vi "Power Supply Control Panel (No Objects).vi"(8 "error in (no error)":errorcluster) -> (0 "error out":errorcluster)   [LabVIEW 2009]
uses:
  Magnet status.ctl
  Oxford/PSSUBS.LLB/PSIO.ctl
  Oxford/BUSGEN.LLB/OxfordAddress.ctl
  Global/Relative Sound Files.vi
  Power Supply.lvclass
panel:
  out "*ips120 (No Ob)":T4={"Field"=0.0, "Rate"=0.0, "Status"={"Sweeping"=FALSE, "Clamped"=FALSE, "Hold"=FALSE, "At Rest"=FALSE, "Quench"=FALSE, "Persistent Mode"=FALSE, "Switch Heater"=FALSE}, "ILM Shut Down?"=FALSE, "IO Info"={"Address"={"Com Port"=1, "ISOBUS Address"=2, "GPIB Address"=24, "Communication"=enum."ISOBUS"}, "Version"=enum."IPS"}, "IO Info (Level Meter)"={"Address"={"Com Port"=1, "ISOBUS Address"=5, "GPIB Address"=24, "Communication"=enum."ISOBUS"}, "ILM Name"="", "Display Channel"=[]}, "Training?"=FALSE, "Training Field and Speed Cluster"={"Training Field"=[0.0, 4.108, 5.78, 8.001], "Training Speed"=[0.0057, 0.0022833333333333334, 0.0011333333333333334, 0.0011333333333333334]}}
  in  "Cluster In":T4={"Field"=0.0, "Rate"=0.0, "Status"={"Sweeping"=FALSE, "Clamped"=FALSE, "Hold"=FALSE, "At Rest"=FALSE, "Quench"=FALSE, "Persistent Mode"=FALSE, "Switch Heater"=FALSE}, "ILM Shut Down?"=FALSE, "IO Info"={"Address"={"Com Port"=1, "ISOBUS Address"=2, "GPIB Address"=24, "Communication"=enum."ISOBUS"}, "Version"=enum."IPS"}, "IO Info (Level Meter)"={"Address"={"Com Port"=1, "ISOBUS Address"=5, "GPIB Address"=24, "Communication"=enum."ISOBUS"}, "ILM Name"="", "Display Channel"=[]}, "Training?"=FALSE, "Training Field and Speed Cluster"={"Training Field"=[0.0, 4.108, 5.78, 8.001], "Training Speed"=[0.0057, 0.0022833333333333334, 0.0011333333333333334, 0.0011333333333333334]}}
  out "Was at persistent?":bool
  in  "Return to persistent?":bool
  out "log counter":dbl
  out "Going to Field?":bool
  out "Current Field":dbl[unit]
  out "Update UI":bool
  out "Status":T1
  in  "Abort Field Sweep":bool
  out "done?":bool
  out "ILM Shut Down?":bool
  out "SH On":bool caption="Switch Heater"
  out "Persistent Mode":bool
  in  "SHcontrol":bool caption="Switch Heater"
  in  "gotopersistent":bool
  out "active":bool
  in  "Train\nMagnet":bool
  out "Busy":bool
  out "ready?":bool
  in  "rate":dbl[unit]=0.016666666666666666 caption="Rate" min=0.0 max=0.25
  in  "Goto":dbl[unit]
  in  "Clamp":bool
  in  "Check for Magnet":bool
  in  "Hold":bool
  in  "Goto Zero":bool
  in  "Goto Field":bool
  in  "endprgm":bool
  # "Magnet Control Panel"
  # "(at current field)"
  # "Off"
  # "On"
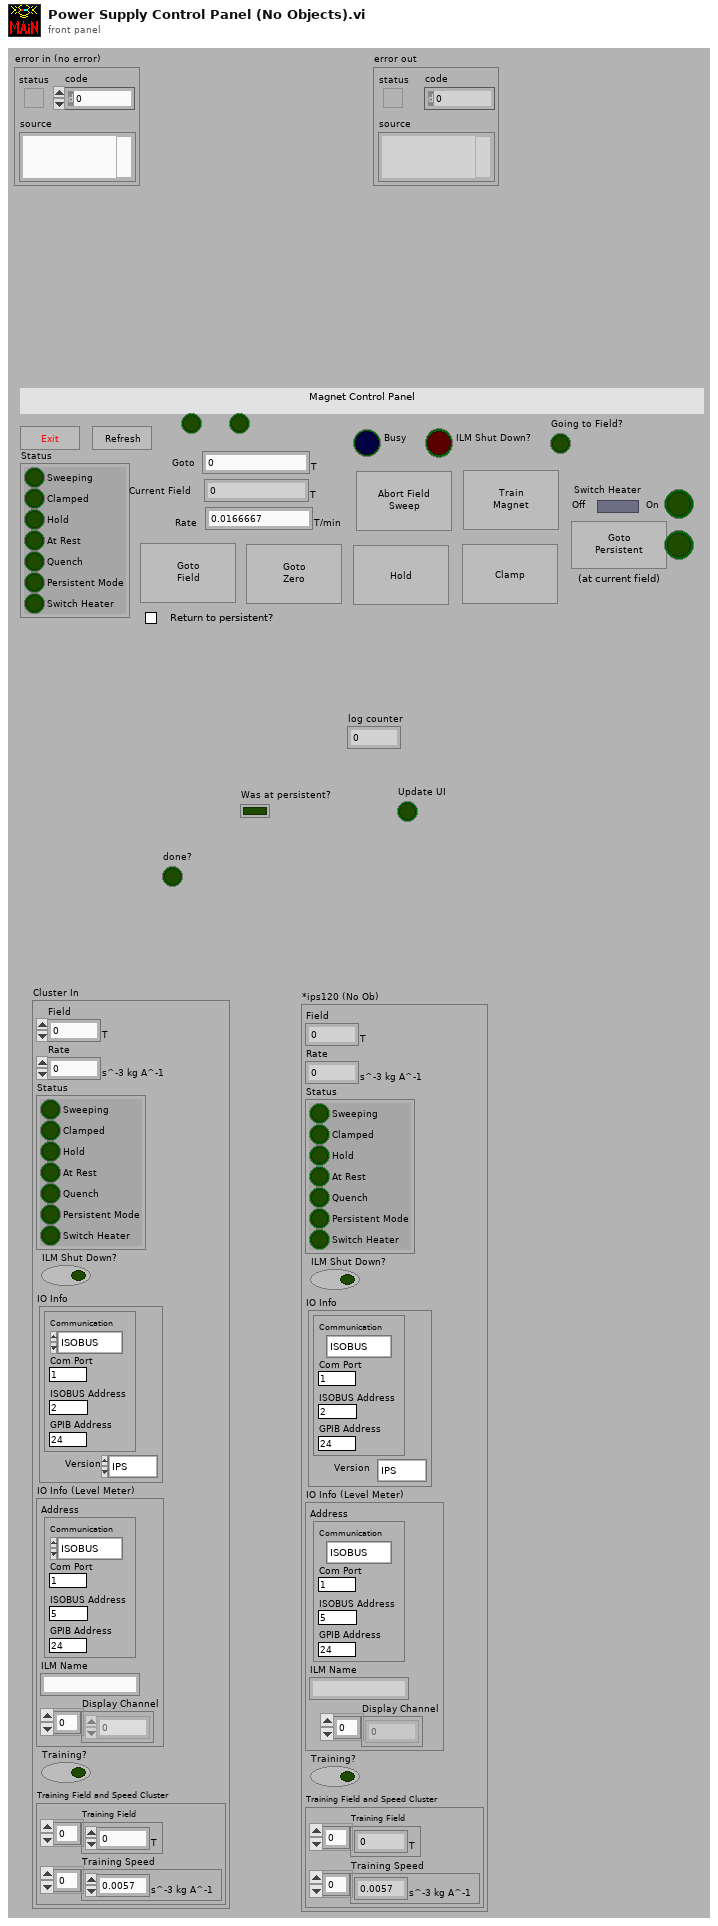
[diagram p1: front panel]
types:
  T1 = typedef "Power Supply.lvclass/Magnet status.ctl" = cluster{"Sweeping":bool, "Clamped":bool, "Hold":bool, "At Rest":bool, "Quench":bool, "Persistent Mode":bool, "Switch Heater":bool}
  T2 = typedef "PSIO.ctl" = cluster{"Address":T3, "Version":enum16{"PS", "IPS"}}
  T3 = typedef "OxfordAddress.ctl" = cluster{"Com Port":i32, "ISOBUS Address":i32, "GPIB Address":i16, "Communication":enum16{"RS232", "ISOBUS", "GPIB", "Gateway"}}
  T4 = cluster{"Field":dbl[unit], "Rate":dbl[unit], "Status":T1, "ILM Shut Down?":bool, "IO Info":T2, "IO Info (Level Meter)":cluster{"Address":T3, "ILM Name":string, "Display Channel":i32[]}, "Training?":bool, "Training Field and Speed Cluster":cluster{"Training Field":dbl[unit][], "Training Speed":dbl[unit][]}}
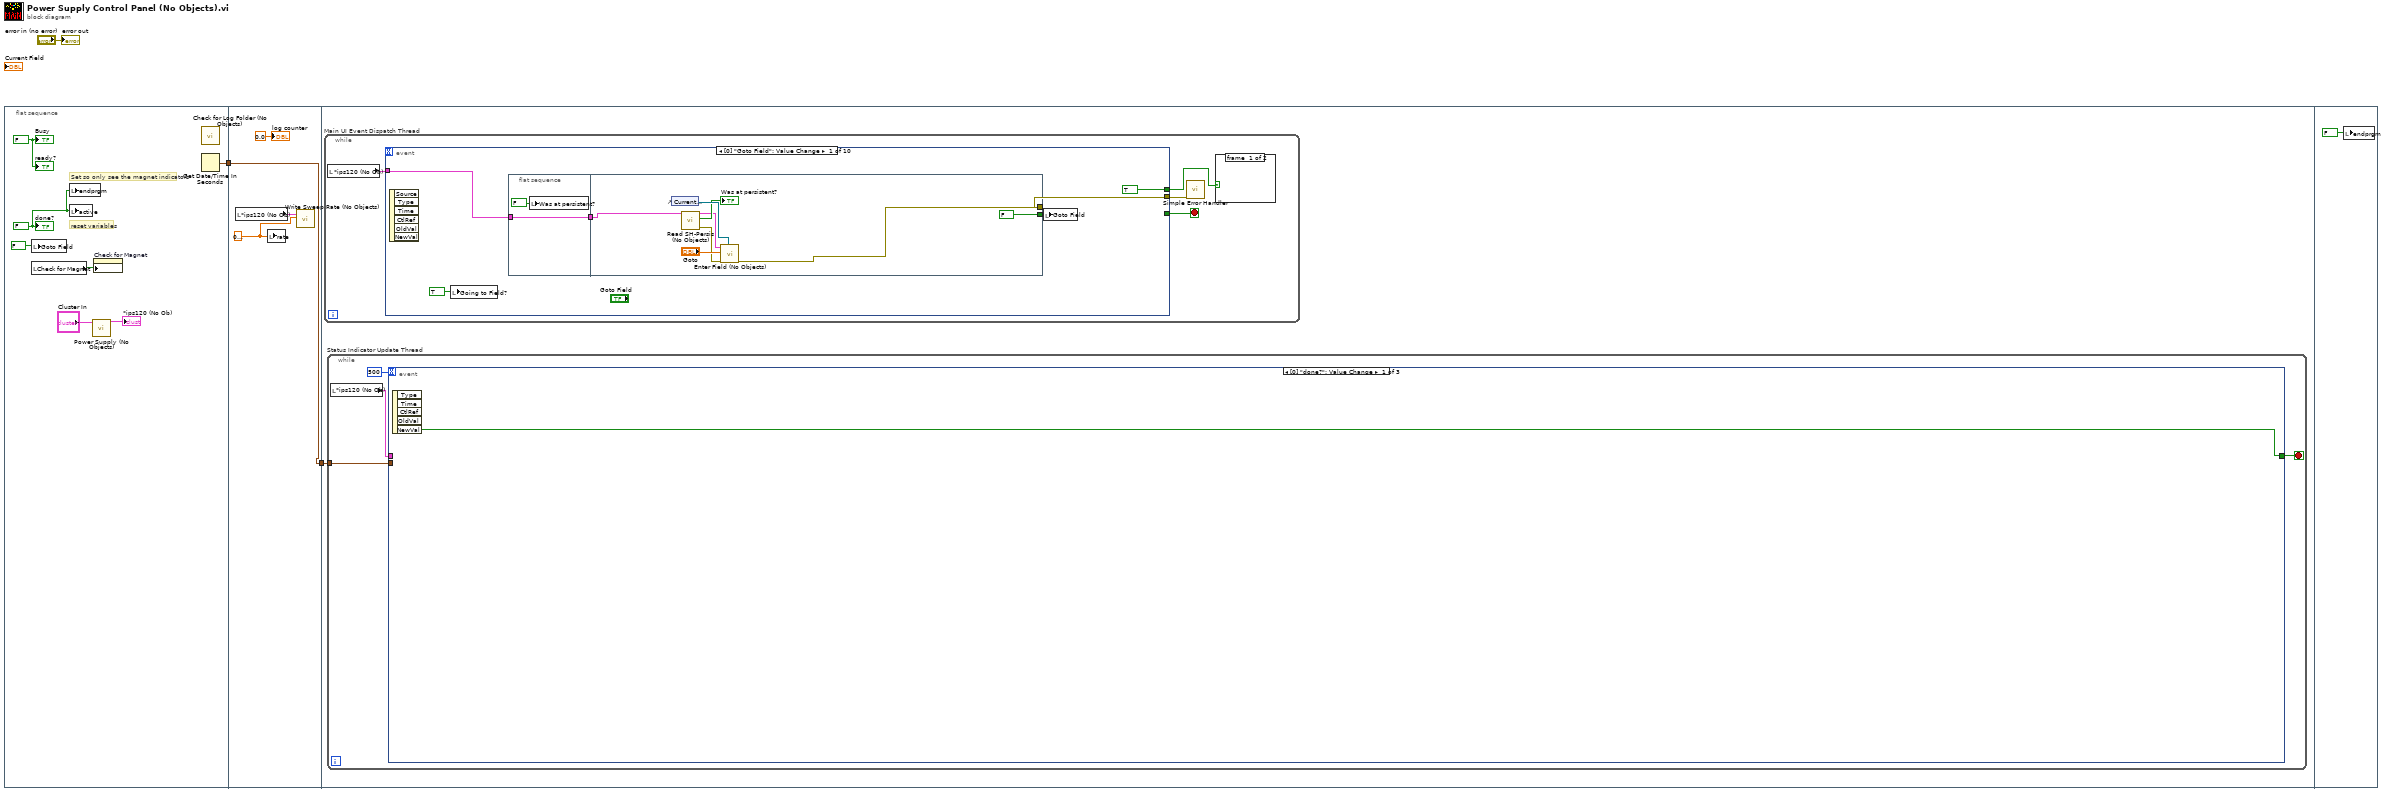
[diagram p0: block diagram]
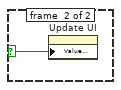
[diagram p2: hidden frame]
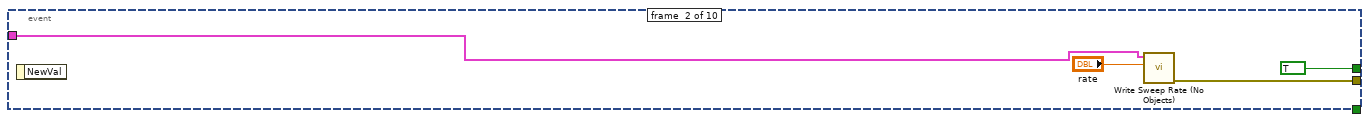
[diagram p3: hidden frame]
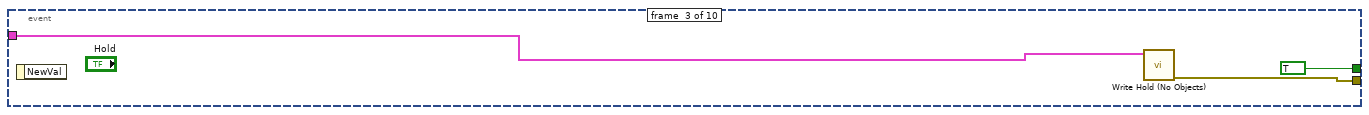
[diagram p4: hidden frame]
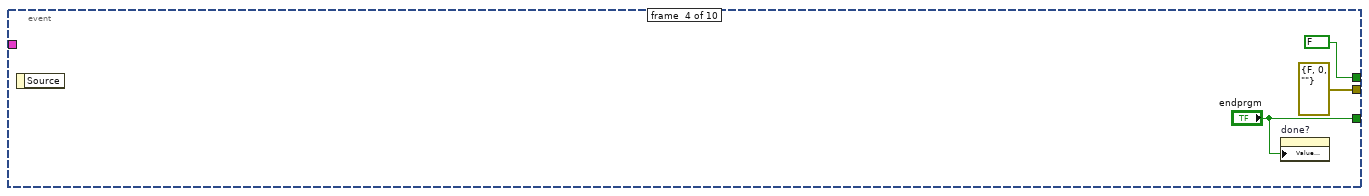
[diagram p5: hidden frame]
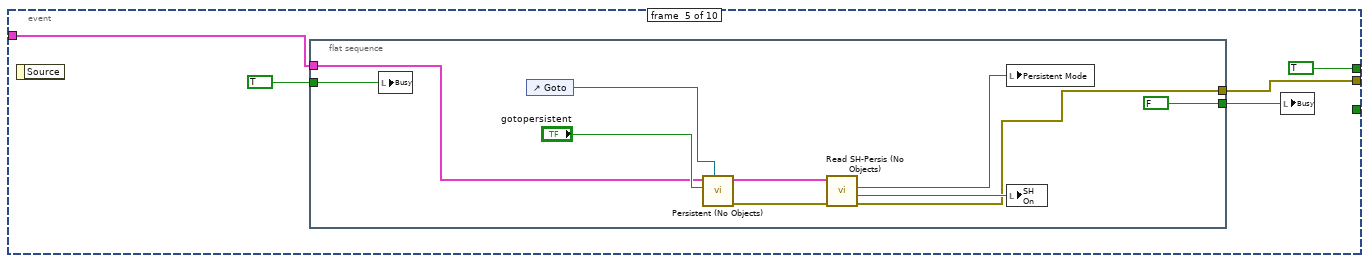
[diagram p6: hidden frame]
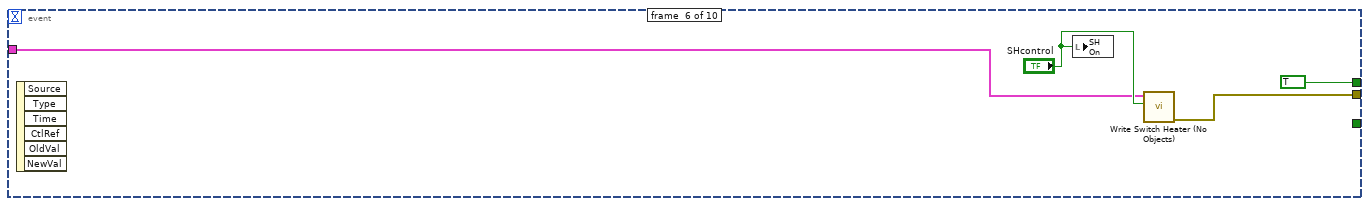
[diagram p7: hidden frame]
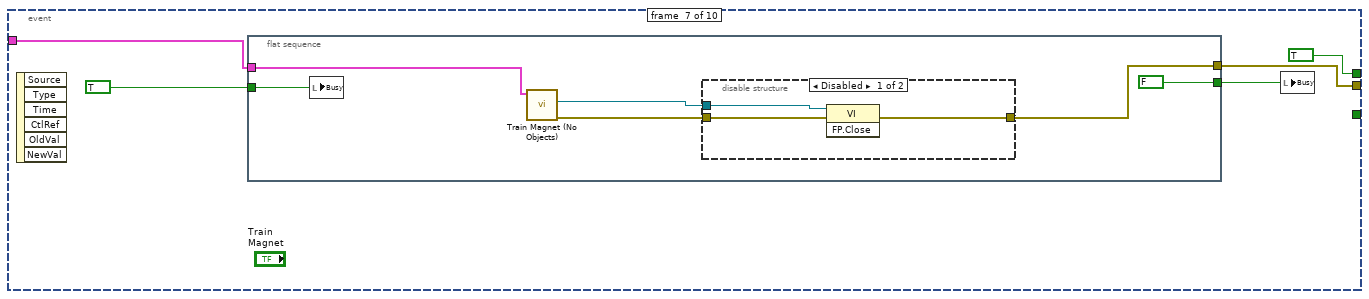
[diagram p8: hidden frame]
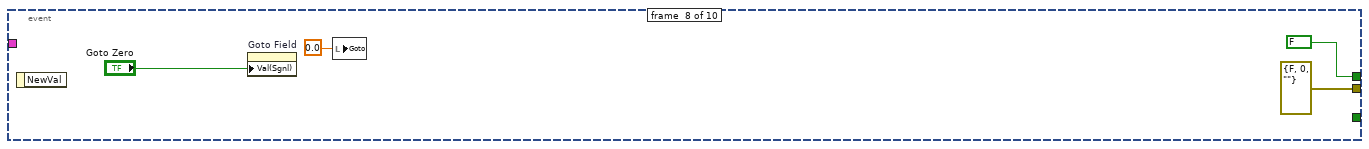
[diagram p10: hidden frame]
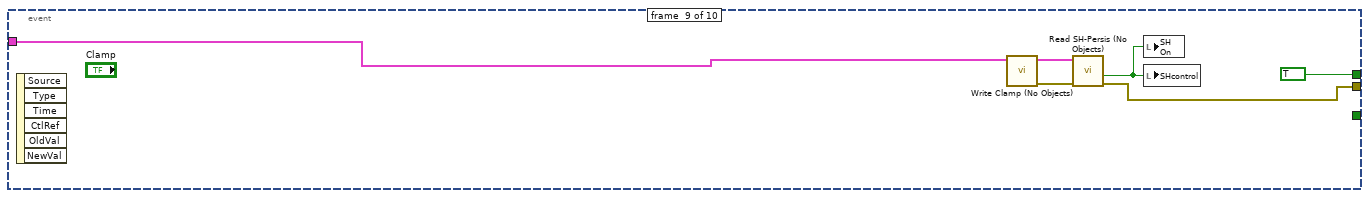
[diagram p11: hidden frame]
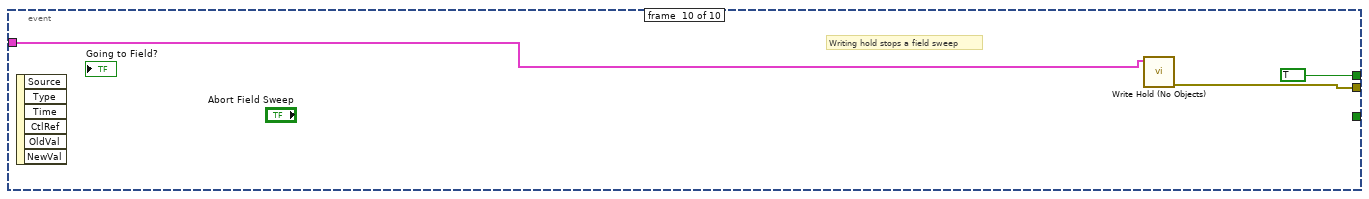
[diagram p12: hidden frame]
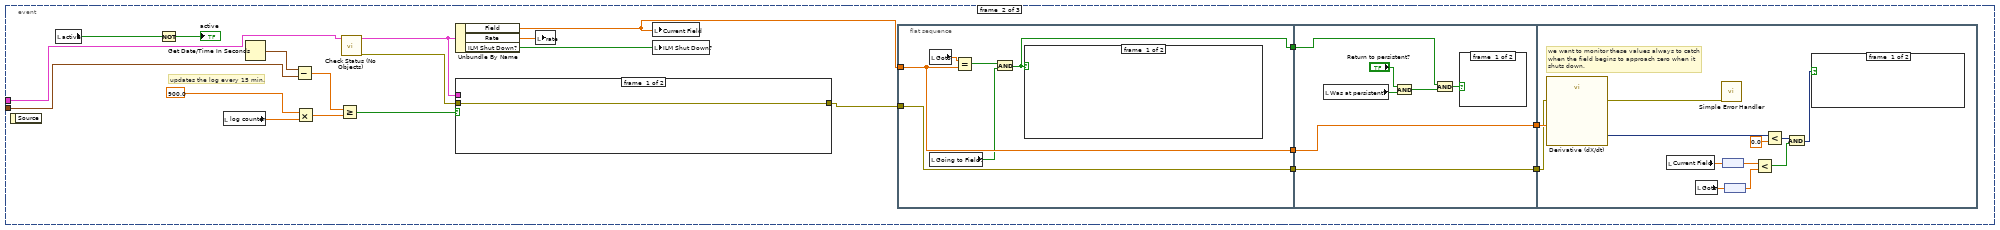
[diagram p13: hidden frame]
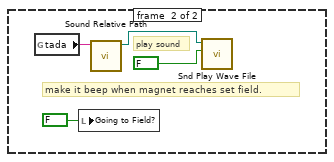
[diagram p14: hidden frame]
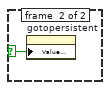
[diagram p15: hidden frame]
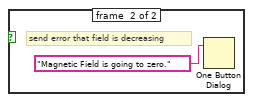
[diagram p16: hidden frame]
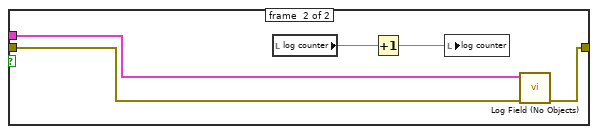
[diagram p17: hidden frame]
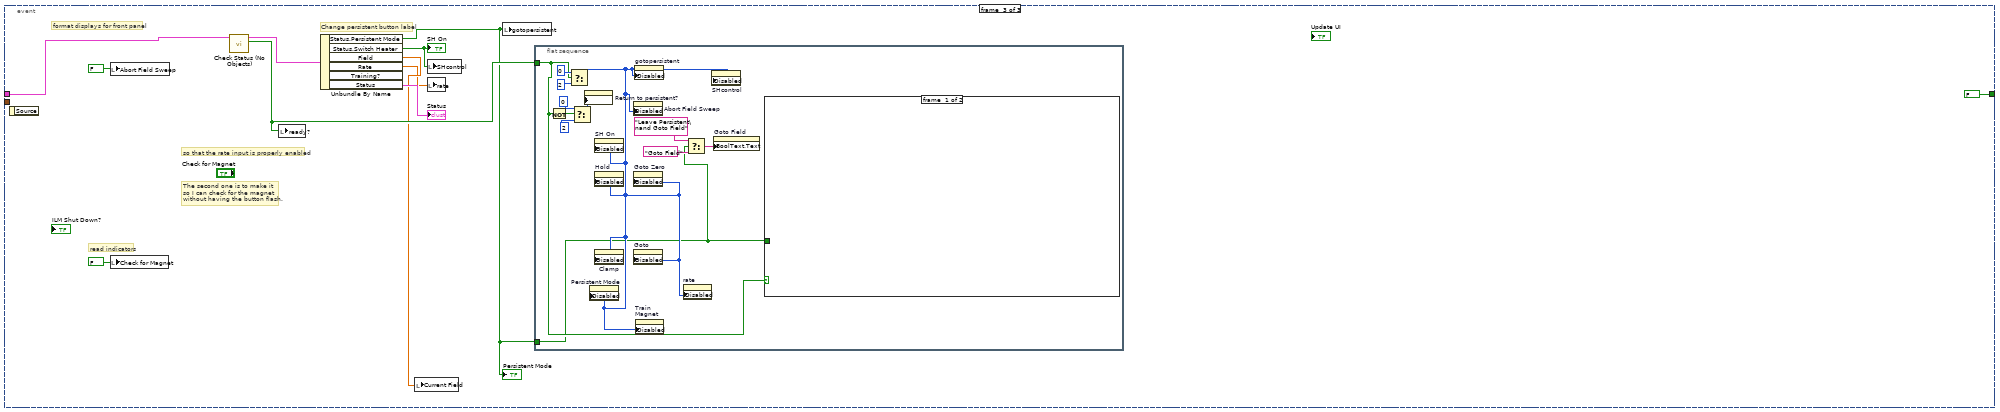
[diagram p18: hidden frame]
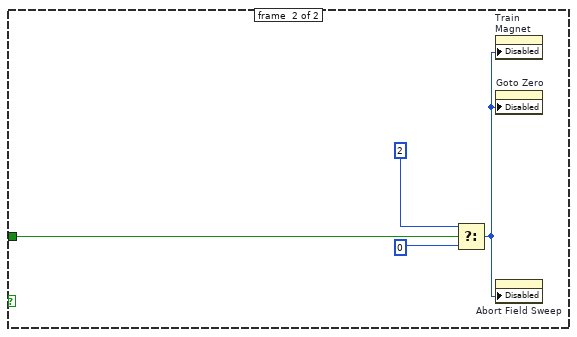
[diagram p19: hidden frame]
diagram:
  n1 = flat-sequence {
    tunnel: [w6] -> w2
    tunnel: w2 -> [w11]
    tunnel: [w11] -> w1
    tunnel: w1 -> [w15]
    frame #0 {
      w10 = FALSE
      w8 = FALSE
      # "Set so only see the magnet indicators"
      # "reset variables"
      n2 = local read "Check for Magnet"() -> (w9:bool)
      n3 = local write "Goto Field"(FALSE ("active")) -> ()
      n4 = local write "endprgm"(w8) -> ()
      n5 = local write "active"(w8) -> ()
      n6 = call "Power Supply (No Objects).vi"("Cluster In"="Cluster In") -> ("Cluster Out"=→"*ips120 (No Ob)":T4)  [unwired: 9 in, 1 out]
      n7 = property on="Check for Magnet" class="Bool (strict)"("Value (Signaling)"=w9) -> ()  [unwired: 2 in, 2 out]
      n8 = call "Check for Log Folder (No Objects).vi"() -> ()  [unwired: 1 in]
      n9 = Get Date/Time In Seconds() -> (seconds since 1Jan1904=w6:timestamp)
      "ready?" <- w10
      "Busy" <- w10
      "done?" <- w8
    }
    frame #1 {
      w12 = dbl[unit] 0.016666666666666666 ("rate")
      n10 = local read "*ips120 (No Ob)"() -> (w13:T4)
      n11 = local write "rate"(w12) -> ()
      n12 = call "Write Sweep Rate (No Objects).vi"("rate"=w12, "Cluster In"=w13) -> ()  [unwired: 8 in, 2 out]
      "log counter" <- 0.0 ("log counter")
    }
    frame #2 {
      n13 = while "Main UI Event Dispatch Thread" {
        stop <- w18 stop-if-true
        n14 = local read "*ips120 (No Ob)"() -> (w16:T4)
        n15 = event shown="[0] \"Goto Field\": Value Change" {
          selector: _ -> [_ _ _ _ _ _ _ _ _ _]
          dyn-events: _ -> [_ _ _ _ _ _ _ _ _ _]
          timeout: _ -> [_ _ _ _ _ _ _ _ _ _]
          tunnel: [_ _ _ "endprgm" _ _ _ _ _ _] -> w18
          tunnel: w16 -> [w26 w38 w41 _ w51 w62 w70 _ w86 w91]
          tunnel: [w24 w37 w42 errorcluster {"status"=FALSE, "code"=0, "source"=""} ("error out") w50 w63 w69 errorcluster {"status"=FALSE, "code"=0, "source"=""} ("error out") w87 w92] -> w19
          tunnel: [TRUE TRUE TRUE FALSE TRUE TRUE TRUE FALSE TRUE TRUE] -> w17
          event #0 {
            n16 = event-data() -> ()  [unwired: 7 out]
            n17 = local write "Going to Field?"(TRUE ("Going to Field?")) -> ()
            n18 = flat-sequence {
              tunnel: w26 -> [w28]
              tunnel: [w28] -> w21
              tunnel: [FALSE ("Goto Field")] -> w25
              tunnel: [w31] -> w24
              tunnel: w21 -> [w30]
              frame #0 {
                n19 = local write "Was at persistent?"(FALSE ("Was at persistent?")) -> ()
              }
              frame #1 {
                n20 = control-ref of="Current Field"() -> (w35:refnum<vi>)
                n21 = call "Read SH-Persis (No Objects).vi"("Cluster In"=w30) -> ("error out"=w33:errorcluster, "pers?"=→"Was at persistent?":bool, "Cluster Out"=w29:T4)  [unwired: 5 in, 3 out]
                n22 = call "Enter Field (No Objects).vi"("Field monitor"=w35, "error in (no error)"=w33, "Target field"="Goto", "Cluster In"=w29) -> ("error out"=w31:errorcluster)  [unwired: 6 in, 1 out]
              }
            }
            n23 = local write "Goto Field"(w25) -> ()
          }
          event #1 {
            n24 = event-data() -> ()  [unwired: 2 out]
            n25 = call "Write Sweep Rate (No Objects).vi"("rate"="rate", "Cluster In"=w38) -> ("error out"=w37:errorcluster)  [unwired: 8 in, 1 out]
          }
          event #2 {
            n26 = event-data() -> ()  [unwired: 2 out]
            n27 = call "Write Hold (No Objects).vi"("Cluster In"=w41) -> ("error out"=w42:errorcluster)  [unwired: 9 in, 1 out]
          }
          event #3 {
            n28 = event-data() -> ()  [unwired: 2 out]
            n29 = property on="done?" class="Boolean (strict)"("Value (Signaling)"="endprgm") -> ()  [unwired: 2 in, 2 out]
          }
          event #4 {
            n30 = event-data() -> ()  [unwired: 2 out]
            n31 = flat-sequence {
              tunnel: w51 -> [w53]
              tunnel: [w54] -> w50
              tunnel: TRUE -> [w56]
              tunnel: [FALSE] -> w47
              frame #0 {
                n32 = local write "Busy"(w56) -> ()
                n33 = control-ref of="Goto"() -> (w60:refnum<vi>)
                n34 = call "Persistent (No Objects).vi"("Field monitor ref"=w60, "Go to persistent mode?"="gotopersistent", "Cluster In"=w53) -> ("error out"=w61:errorcluster, "Cluster Out"=w52:T4)  [unwired: 7 in]
                n35 = call "Read SH-Persis (No Objects).vi"("error in (no error)"=w61, "Cluster In"=w52) -> ("error out"=w54:errorcluster, "SHon?"=w57:bool, "pers?"=w58:bool)  [unwired: 4 in, 3 out]
                n36 = local write "Persistent Mode"(w58) -> ()
                n37 = local write "SH On"(w57) -> ()
              }
            }
            n38 = local write "Busy"(w47) -> ()
          }
          event #5 {
            n39 = event-data() -> ()  [unwired: 7 out]
            n40 = local write "SH On"("SHcontrol") -> ()
            n41 = call "Write Switch Heater (No Objects).vi"("Turn SH On?"="SHcontrol", "Cluster In"=w62) -> ("error out"=w63:errorcluster)  [unwired: 8 in, 1 out]
          }
          event #6 {
            n42 = event-data() -> ()  [unwired: 7 out]
            n43 = flat-sequence {
              tunnel: w70 -> [w71]
              tunnel: [w72] -> w69
              tunnel: [FALSE] -> w67
              tunnel: TRUE -> [w75]
              frame #0 {
                n44 = local write "Busy"(w75) -> ()
                n45 = call "Train Magnet (No Objects).vi"("Cluster In"=w71) -> ("error out"=w73:errorcluster, "This VI"=w74:refnum<vi>)  [unwired: 8 in, 1 out]
                n46 = disable-structure shown="Disabled" {
                  disable-tunnel: w74 -> [w79 _]
                  disable-tunnel: w73 -> [w78 w80]
                  disable-tunnel: [w77 w80] -> w72
                  frame #0 {
                    n47 = invoke class="VI" method="FP.Close"(reference=w79, error in=w78) -> (error out=w77:errorcluster)  [unwired: 1 in, 2 out]
                  }
                  frame #1 {
                  }
                }
              }
            }
            n48 = local write "Busy"(w67) -> ()
          }
          event #7 {
            n49 = event-data() -> ()  [unwired: 2 out]
            n50 = property on="Goto Field" class="Bool (strict)"("Val(Sgnl)"="Goto Zero") -> ()  [unwired: 2 in, 2 out]
            n51 = local write "Goto"(dbl[unit] 0.0 ("Goto")) -> ()
          }
          event #8 {
            n52 = event-data() -> ()  [unwired: 7 out]
            n53 = call "Write Clamp (No Objects).vi"("Cluster In"=w86) -> ("error out"=w90:errorcluster, "Cluster Out"=w85:T4)  [unwired: 9 in]
            n54 = call "Read SH-Persis (No Objects).vi"("error in (no error)"=w90, "Cluster In"=w85) -> ("error out"=w87:errorcluster, "SHon?"=w89:bool)  [unwired: 4 in, 4 out]
            n55 = local write "SH On"(w89) -> ()
            n56 = local write "SHcontrol"(w89) -> ()
          }
          event #9 {
            # "Writing hold stops a field sweep"
            n57 = event-data() -> ()  [unwired: 7 out]
            n58 = call "Write Hold (No Objects).vi"("Cluster In"=w91) -> ("error out"=w92:errorcluster)  [unwired: 9 in, 1 out]
          }
        }
        n59 = call <vilib>:"Simple Error Handler.vi"("error in (no error)"=w19) -> ()  [unwired: 4 in, 5 out]
        n60 = case shown="True" w17 {
          selector: w17 -> [_ w20]
          frame #0 {
          }
          frame #1 {
            n61 = property on="Update UI" class="Bool (strict)"("Value (Signaling)"=w20) -> ()  [unwired: 2 in, 2 out]
          }
        }
      }
      n62 = while "Status Indicator Update Thread" {
        tunnel: w15 -> [w95]
        stop <- w96 stop-if-true
        n63 = local read "*ips120 (No Ob)"() -> (w94:T4)
        n64 = event shown="[0] \"done?\": Value Change" {
          selector: _ -> [_ _ _]
          dyn-events: _ -> [_ _ _]
          timeout: 500 -> [_ _ _]
          tunnel: [w98 _ FALSE] -> w96
          tunnel: w94 -> [_ w100 w157]
          tunnel: w95 -> [_ w117 _]
          event #0 {
            n65 = event-data() -> ("NewVal"=w98:bool)  [unwired: 5 out]
          }
          event #1 {
            # "updates the log every 15 min."
            n66 = event-data() -> ()  [unwired: 2 out]
            n67 = local read "active"() -> (w119:bool)
            n68 = Not(x=w119) -> (.not. x?=→"active":bool)
            n69 = local read "log counter"() -> (w108:dbl)
            n70 = Get Date/Time In Seconds() -> (seconds since 1Jan1904=w111:timestamp)
            n71 = Subtract(x=w111, y=w117) -> (x-y=w106:dbl)
            n72 = Multiply(x=900.0 ("millisecond multiple"), y=w108) -> (x*y=w107:dbl)
            n73 = Greater Or Equal?(x=w106, y=w107) -> (x >= y?=w112:bool)
            n74 = call "Check Status (No Objects).vi"("Cluster In"=w100) -> ("error out"=w113:errorcluster, "Cluster Out"=w114:T4)  [unwired: 7 in, 2 out]
            n75 = Unbundle By Name(w114) -> ("Field"=w115:dbl[unit], "Rate"=w110:dbl[unit], "ILM Shut Down?"=w116:bool)
            n76 = case shown="True" w112 {
              tunnel: [w151 w156] -> w99
              tunnel: w114 -> [_ w152]
              tunnel: w113 -> [w151 w155]
              frame #0 {
              }
              frame #1 {
                n77 = local read "log counter"() -> (w154:dbl)
                n78 = Increment(x=w154) -> (x+1=w153:dbl)
                n79 = local write "log counter"(w153) -> ()
                n80 = call "Log Field (No Objects).vi"("error in (no error)"=w155, "Cluster In"=w152) -> ("error out"=w156:errorcluster)  [unwired: 8 in, 1 out]
              }
            }
            n81 = local write "rate"(w110) -> ()
            n82 = local write "Current Field"(w115) -> ()
            n83 = local write "ILM Shut Down?"(w116) -> ()
            n84 = flat-sequence {
              tunnel: w99 -> [w125]
              tunnel: w115 -> [w123]
              tunnel: [w123] -> w105
              tunnel: [w125] -> w104
              tunnel: [w120] -> w103
              tunnel: w105 -> [w136]
              tunnel: [w136] -> w102
              tunnel: w104 -> [w135]
              tunnel: [w135] -> w101
              tunnel: w103 -> [w133]
              tunnel: w102 -> [w149]
              tunnel: w101 -> [w148]
              frame #0 {
                n85 = local read "Goto"() -> (w124:dbl[unit])
                n86 = local read "Going to Field?"() -> (w121:bool)
                n87 = Equal?(x=w124, y=w123) -> (x = y?=w122:bool)
                n88 = And(x=w122, y=w121) -> (x .and. y?=w120:bool)
                n89 = case shown="True" w120 {
                  frame #0 {
                  }
                  frame #1 {
                    # "make it beep when magnet reaches set field."
                    # "play sound"
                    n90 = global read "Relative Sound Files.vi" "tada"() -> (w127:string)
                    n91 = local write "Going to Field?"(FALSE ("Going to Field?")) -> ()
                    n92 = call "Sound Relative Path.vi"("Sound"=w127) -> ("Relative Path"=w128:path)  [unwired: 10 in]
                    n93 = call <vilib>:"Snd Play Wave File.vi"("wait until finish (T)"=FALSE, "wave file path"=w128) -> ()  [unwired: 1 in, 9 out]
                  }
                }
              }
              frame #1 {
                n94 = local read "Was at persistent?"() -> (w132:bool)
                n95 = And(x="Return to persistent?", y=w132) -> (x .and. y?=w130:bool)
                n96 = And(x=w133, y=w130) -> (x .and. y?=w134:bool)
                n97 = case shown="True" w134 {
                  selector: w134 -> [_ w137]
                  frame #0 {
                  }
                  frame #1 {
                    n98 = property on="gotopersistent" class="Bool (strict)"("Value (Signaling)"=w137) -> ()  [unwired: 2 in, 2 out]
                  }
                }
              }
              frame #2 {
                # "we want to monitor these values always to catch\nwhen the field begins to approach zero when it\nshuts down."
                n99 = call "Derivative (dX/dt)"("error in (no error)"=w148, "Signals"=w149) -> ("error out"=w143:errorcluster, "Result"=w147:dynamicdata)  [unwired: 4 out]
                n100 = local read "Current Field"() -> (w139:dbl[unit])
                n101 = local read "Goto"() -> (w141:dbl[unit])
                n102 = call <vilib>:"Simple Error Handler.vi"("error in (no error)"=w143) -> ()  [unwired: 4 in, 5 out]
                n103 = node(w139) -> (w138:dbl)
                n104 = node(w141) -> (w140:dbl)
                n105 = Less?(x=w138, y=w140) -> (x < y?=w142:bool)
                n106 = Less?(x=w147, y=0.0) -> (x < y?=w145:dynamicdata)
                n107 = And(x=w145, y=w142) -> (x .and. y?=w144:dynamicdata)
                n108 = case shown="True" w144 {
                  frame #0 {
                  }
                  frame #1 {
                    # "send error that field is decreasing"
                    n109 = One Button Dialog(message="Magnetic Field is going to zero.") -> ()  [unwired: 1 in, 1 out]
                  }
                }
              }
            }
          }
          event #2 {
            # "format displays for front panel"
            # "read indicators"
            # "so that the rate input is properly enabled"
            # "Change persistent button label"
            # "The second one is to make it\nso I can check for the magnet\nwithout having the button flash."
            n110 = event-data() -> ()  [unwired: 2 out]
            n111 = local write "Abort Field Sweep"(FALSE ("Abort Field Sweep")) -> ()
            n112 = local write "Check for Magnet"(FALSE) -> ()
            n113 = call "Check Status (No Objects).vi"("Cluster In"=w157) -> ("Ready?"=w165:bool, "Cluster Out"=w163:T4)  [unwired: 7 in, 2 out]
            n114 = local write "ready?"(w165) -> ()
            n115 = Unbundle By Name(w163) -> ("Status.Persistent Mode"=w160:bool, "Status.Switch Heater"=w164:bool, "Field"=w161:dbl[unit], "Rate"=w158:dbl[unit], "Status"=→"Status":T1)  [unwired: 1 out]
            "Persistent Mode" <- w160
            "SH On" <- w164
            n116 = local write "Current Field"(w161) -> ()
            n117 = local write "SHcontrol"(w164) -> ()
            n118 = local write "rate"(w158) -> ()
            n119 = local write "gotopersistent"(w160) -> ()
            n120 = flat-sequence {
              tunnel: w160 -> [w168]
              tunnel: w165 -> [w174]
              frame #0 {
                n121 = Not(x=w174) -> (.not. x?=w173:bool)
                n122 = Select(t=0, s=w174, f=2) -> (s? t:f=w177:i32)
                n123 = Select(t=0, s=w173, f=2) -> (s? t:f=w172:i32)
                n124 = property on="Return to persistent?" class="Bool (strict)"("DisabledEnum"=w172) -> ()  [unwired: 2 in, 2 out]
                n125 = property on="Persistent Mode" class="Boolean (strict)"("Disabled"=w177) -> ()  [unwired: 2 in, 2 out]
                n126 = property on="SH On" class="Boolean (strict)"("Disabled"=w177) -> ()  [unwired: 2 in, 2 out]
                n127 = property on="Hold" class="Boolean"("Disabled"=w177) -> ()  [unwired: 2 in, 2 out]
                n128 = property on="Clamp" class="Boolean"("Disabled"=w177) -> ()  [unwired: 2 in, 2 out]
                n129 = property on="Abort Field Sweep" class="Bool (strict)"("Disabled"=w177) -> ()  [unwired: 2 in, 2 out]
                n130 = property on="Goto Zero" class="Bool"("Disabled"=w177) -> ()  [unwired: 2 in, 2 out]
                n131 = property on="Goto" class="DigNum (strict)"("Disabled"=w177) -> ()  [unwired: 2 in, 2 out]
                n132 = property on="gotopersistent" class="Bool (strict)"("Disabled"=w177) -> ()  [unwired: 2 in, 2 out]
                n133 = property on="Train\nMagnet" class="Boolean"("Disabled"=w177) -> ()  [unwired: 2 in, 2 out]
                n134 = property on="rate" class="DigNum (strict)"("Disabled"=w177) -> ()  [unwired: 2 in, 2 out]
                n135 = Select(t="Leave Persistent\nand Goto Field", s=w168, f="Goto Field") -> (s? t:f=w170:string)
                n136 = property on="SHcontrol" class="Boolean (strict)"("Disabled"=w177) -> ()  [unwired: 2 in, 2 out]
                n137 = property on="Goto Field" class="Bool (strict)"("BoolText.Text"=w170) -> ()  [unwired: 2 in, 2 out]
                n138 = case shown="True" w174 {
                  tunnel: w168 -> [_ w181]
                  frame #0 {
                  }
                  frame #1 {
                    n139 = Select(t=2, s=w181, f=0) -> (s? t:f=w180:i32)
                    n140 = property on="Train\nMagnet" class="Boolean"("Disabled"=w180) -> ()  [unwired: 2 in, 2 out]
                    n141 = property on="Goto Zero" class="Bool"("Disabled"=w180) -> ()  [unwired: 2 in, 2 out]
                    n142 = property on="Abort Field Sweep" class="Bool (strict)"("Disabled"=w180) -> ()  [unwired: 2 in, 2 out]
                  }
                }
              }
            }
          }
        }
      }
    }
    frame #3 {
      n143 = local write "endprgm"(FALSE) -> ()
    }
  }
  "error out" <- "error in (no error)"
